vi "Update.vi"(0 "Interface In":refnum<class "VdLaser_MyINterface.lvclass">, 5 "error in (no error)":errorcluster) -> (14 "Interface Out":refnum<class "VdLaser_MyINterface.lvclass">, 19 "error out":errorcluster)   [LabVIEW 2010, in "VdLaser_MyINterface.lvclass"]
uses:
  VdLaser_MyINterface.lvclass
  VdLaser_MyINterface.lvclass/VdLaser_MyINterface.ctl
  VdLaser_class/VdLaser.lvclass
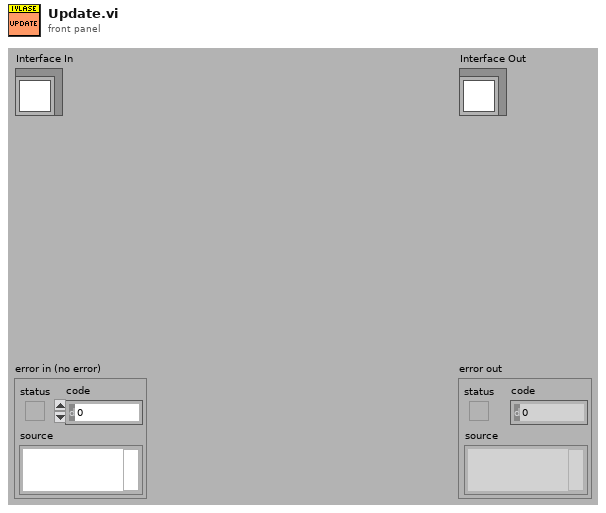
[diagram p1: front panel]
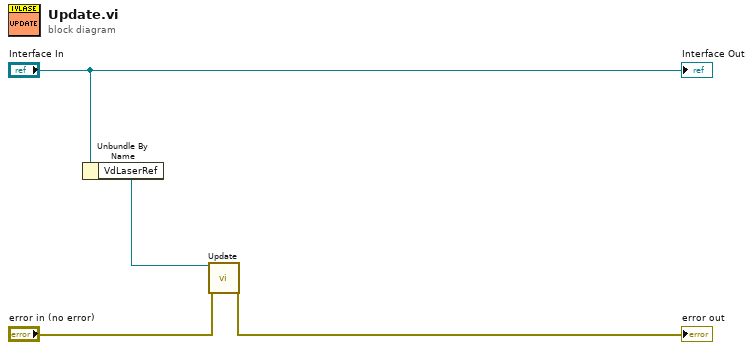
[diagram p0: block diagram]
diagram:
  n1 = Unbundle By Name("Interface In") -> ("VdLaserRef"=w1:refnum<class "VdLaser.lvclass">)
  n2 = call-dynamic "Update.vi"("reference in"=w1, "error in (no error)"="error in (no error)") -> ("error out"=→"error out":errorcluster)  [unwired: 16 in, 1 out]
  "Interface Out" <- "Interface In"
